vi "JSONRPC-BuildParam.vi"(8 "Value":string, 9 "Location":string, 10 "Required":bool, 11 "Name":string) -> (3 "Output":string)   [LabVIEW 2015]
panel:
  # "BuildParam"
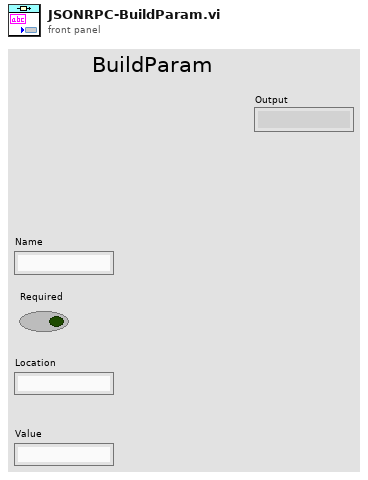
[diagram p1: front panel]
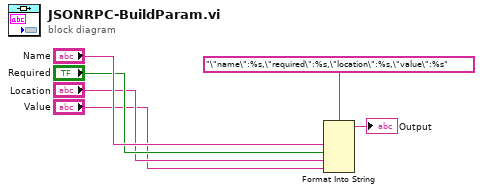
[diagram p0: block diagram]
diagram:
  n1 = Format Into String(format string="\"name\":%s,\"required\":%s,\"location\":%s,\"value\":%s", "Name", "Required", "Location", "Value") -> (resulting string=→"Output":string)  [unwired: 2 in, 1 out]
